vi "SRU（I16）.vi"(6 "复位":bool, 9 "初始值":i16, 10 "输入":i16) -> (1 "本次值":i16, 2 "上次值":i16, 5 "初始值":i16)   [LabVIEW 2013, in "寄存器单元SRU.lvlib"]
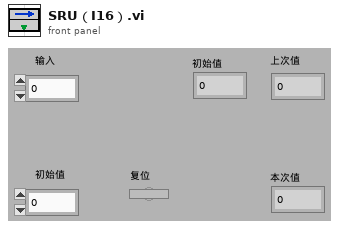
[diagram p1: front panel]
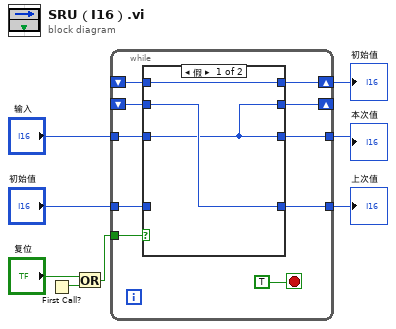
[diagram p0: block diagram]
diagram:
  n1 = First Call?() -> (First Call?: T/F=w7:bool)
  n2 = Or(x="复位", y=w7) -> (x .or. y?=w6:bool)
  n3 = while {
    tunnel: w6 -> [w17]
    shift-right: [w15] -> w2
    shift-left: _ -> [w13]
    shift-right: [w14] -> _
    shift-left: _ -> [w11]
    tunnel: "初始值" -> [w16]
    tunnel: "输入" -> [w12]
    tunnel: [w10] -> w3
    tunnel: [w9] -> w1
    stop <- TRUE stop-if-true
    n4 = case shown="假" w17 {
      tunnel: w16 -> [_ w23]
      tunnel: [w21 w23] -> w15
      tunnel: [w19 w23] -> w14
      tunnel: w13 -> [w21 _]
      tunnel: w12 -> [w19 w22]
      tunnel: w11 -> [w20 _]
      tunnel: [w20 w23] -> w10
      tunnel: [w19 w22] -> w9
      frame False {
      }
      frame True {
      }
    }
  }
  "上次值" <- w3
  "初始值" <- w2
  "本次值" <- w1
